vi "WKLXF25 Get Part Information 3.0.vi"(8 "error in":errorcluster, 11 "PLC Tags":T2={"Serial Number"={"Tag Name"="S060.PXI.Signals.PlltData.SN", "Network Path"="172.15.51.1,1,0", "use opc"=FALSE, "DataSocket Reference"={"CWDSLib._DCWDataSocket"=refnum, "CWDSLib._DCWData"=refnum, "OnDataUpdated"=0, "OnStatusUpdated"=0}}, "Pallet Number"={"Tag Name"="S060.PXI.Signals.PlltData.SN", "Network Path"="172.15.51.1,1,0", "use opc"=FALSE, "DataSocket Reference"={"CWDSLib._DCWDataSocket"=refnum, "CWDSLib._DCWData"=refnum, "OnDataUpdated"=0, "OnStatusUpdated"=0}}, "Inalfa Part Number"={"Tag Name"="S060.PXI.Signals.PlltData.SN", "Network Path"="172.15.51.1,1,0", "use opc"=FALSE, "DataSocket Reference"={"CWDSLib._DCWDataSocket"=refnum, "CWDSLib._DCWData"=refnum, "OnDataUpdated"=0, "OnStatusUpdated"=0}}, "Shade Color"={"Tag Name"="S060.PXI.Signals.PlltData.SN", "Network Path"="172.15.51.1,1,0", "use opc"=FALSE, "DataSocket Reference"={"CWDSLib._DCWDataSocket"=refnum, "CWDSLib._DCWData"=refnum, "OnDataUpdated"=0, "OnStatusUpdated"=0}}, "Model Type"={"Tag Name"="S060.PXI.Signals.PlltData.SN", "Network Path"="172.15.51.1,1,0", "use opc"=FALSE, "DataSocket Reference"={"CWDSLib._DCWDataSocket"=refnum, "CWDSLib._DCWData"=refnum, "OnDataUpdated"=0, "OnStatusUpdated"=0}}, "Customer Number"={"Tag Name"="S060.PXI.Signals.PlltData.SN", "Network Path"="172.15.51.1,1,0", "use opc"=FALSE, "DataSocket Reference"={"CWDSLib._DCWDataSocket"=refnum, "CWDSLib._DCWData"=refnum, "OnDataUpdated"=0, "OnStatusUpdated"=0}}, "Part History Number"={"Tag Name"="S060.PXI.Signals.PlltData.SN", "Network Path"="172.15.51.1,1,0", "use opc"=FALSE, "DataSocket Reference"={"CWDSLib._DCWDataSocket"=refnum, "CWDSLib._DCWData"=refnum, "OnDataUpdated"=0, "OnStatusUpdated"=0}}, "Shade 1 Barcode"={"Tag Name"="S060.PXI.Signals.PlltData.SN", "Network Path"="172.15.51.1,1,0", "use opc"=FALSE, "DataSocket Reference"={"CWDSLib._DCWDataSocket"=refnum, "CWDSLib._DCWData"=refnum, "OnDataUpdated"=0, "OnStatusUpdated"=0}}, "Shade 2 Barcode"={"Tag Name"="S060.PXI.Signals.PlltData.SN", "Network Path"="172.15.51.1,1,0", "use opc"=FALSE, "DataSocket Reference"={"CWDSLib._DCWDataSocket"=refnum, "CWDSLib._DCWData"=refnum, "OnDataUpdated"=0, "OnStatusUpdated"=0}}, "Manual Serial Number"={"Tag Name"="S060.PXI.Signals.PlltData.SN", "Network Path"="172.15.51.1,1,0", "use opc"=FALSE, "DataSocket Reference"={"CWDSLib._DCWDataSocket"=refnum, "CWDSLib._DCWData"=refnum, "OnDataUpdated"=0, "OnStatusUpdated"=0}}, "Manual Inalfa Part Number"={"Tag Name"="S060.PXI.Signals.PlltData.SN", "Network Path"="172.15.51.1,1,0", "use opc"=FALSE, "DataSocket Reference"={"CWDSLib._DCWDataSocket"=refnum, "CWDSLib._DCWData"=refnum, "OnDataUpdated"=0, "OnStatusUpdated"=0}}, "Manual Shade Color"={"Tag Name"="S060.PXI.Signals.PlltData.SN", "Network Path"="172.15.51.1,1,0", "use opc"=FALSE, "DataSocket Reference"={"CWDSLib._DCWDataSocket"=refnum, "CWDSLib._DCWData"=refnum, "OnDataUpdated"=0, "OnStatusUpdated"=0}}, "Manual Model Type"={"Tag Name"="S060.PXI.Signals.PlltData.SN", "Network Path"="172.15.51.1,1,0", "use opc"=FALSE, "DataSocket Reference"={"CWDSLib._DCWDataSocket"=refnum, "CWDSLib._DCWData"=refnum, "OnDataUpdated"=0, "OnStatusUpdated"=0}}, "Manual Customer Number"={"Tag Name"="S060.PXI.Signals.PlltData.SN", "Network Path"="172.15.51.1,1,0", "use opc"=FALSE, "DataSocket Reference"={"CWDSLib._DCWDataSocket"=refnum, "CWDSLib._DCWData"=refnum, "OnDataUpdated"=0, "OnStatusUpdated"=0}}, "Manual Part History Number"={"Tag Name"="S060.PXI.Signals.PlltData.SN", "Network Path"="172.15.51.1,1,0", "use opc"=FALSE, "DataSocket Reference"={"CWDSLib._DCWDataSocket"=refnum, "CWDSLib._DCWData"=refnum, "OnDataUpdated"=0, "OnStatusUpdated"=0}}} {"Manual Part History Number"."DataSocket Reference"."OnStatusUpdated" format="%.0x"; "Manual Part History Number"."DataSocket Reference"."OnDataUpdated" format="%.0x"; "Manual Customer Number"."DataSocket Reference"."OnStatusUpdated" format="%.0x"; "Manual Customer Number"."DataSocket Reference"."OnDataUpdated" format="%.0x"; "Manual Model Type"."DataSocket Reference"."OnStatusUpdated" format="%.0x"; "Manual Model Type"."DataSocket Reference"."OnDataUpdated" format="%.0x"; "Manual Shade Color"."DataSocket Reference"."OnStatusUpdated" format="%.0x"; "Manual Shade Color"."DataSocket Reference"."OnDataUpdated" format="%.0x"; "Manual Inalfa Part Number"."DataSocket Reference"."OnStatusUpdated" format="%.0x"; "Manual Inalfa Part Number"."DataSocket Reference"."OnDataUpdated" format="%.0x"; "Manual Serial Number"."DataSocket Reference"."OnStatusUpdated" format="%.0x"; "Manual Serial Number"."DataSocket Reference"."OnDataUpdated" format="%.0x"; "Shade 2 Barcode"."DataSocket Reference"."OnStatusUpdated" format="%.0x"; "Shade 2 Barcode"."DataSocket Reference"."OnDataUpdated" format="%.0x"; "Shade 1 Barcode"."DataSocket Reference"."OnStatusUpdated" format="%.0x"; "Shade 1 Barcode"."DataSocket Reference"."OnDataUpdated" format="%.0x"; "Part History Number"."DataSocket Reference"."OnStatusUpdated" format="%.0x"; "Part History Number"."DataSocket Reference"."OnDataUpdated" format="%.0x"; "Customer Number"."DataSocket Reference"."OnStatusUpdated" format="%.0x"; "Customer Number"."DataSocket Reference"."OnDataUpdated" format="%.0x"; "Model Type"."DataSocket Reference"."OnStatusUpdated" format="%.0x"; "Model Type"."DataSocket Reference"."OnDataUpdated" format="%.0x"; "Shade Color"."DataSocket Reference"."OnStatusUpdated" format="%.0x"; "Shade Color"."DataSocket Reference"."OnDataUpdated" format="%.0x"; "Inalfa Part Number"."DataSocket Reference"."OnStatusUpdated" format="%.0x"; "Inalfa Part Number"."DataSocket Reference"."OnDataUpdated" format="%.0x"; "Pallet Number"."DataSocket Reference"."OnStatusUpdated" format="%.0x"; "Pallet Number"."DataSocket Reference"."OnDataUpdated" format="%.0x"; "Serial Number"."DataSocket Reference"."OnStatusUpdated" format="%.0x"; "Serial Number"."DataSocket Reference"."OnDataUpdated" format="%.0x"}) -> (0 "error out":errorcluster, 2 "Good Data?":bool, 3 "part info":T1)   [LabVIEW 2018]
uses:
  02.Type Def's/station plc read string tags.ctl
  05.UserVI's/type defs/plc path and tag.ctl
  <vilib>/Platform/dataskt.llb/DataSocket Reference Type.ctl
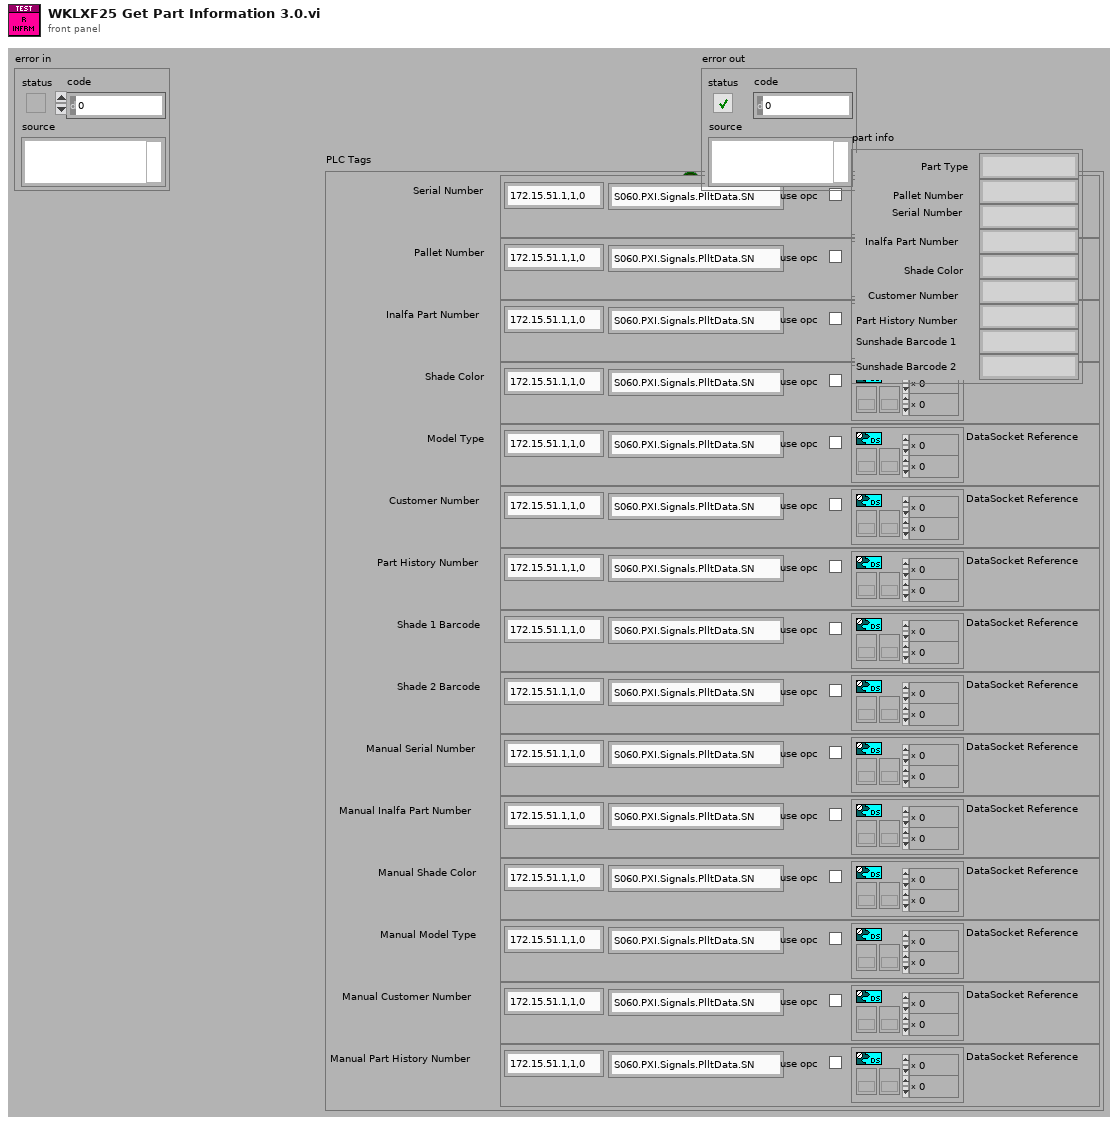
[diagram p1: front panel]
types:
  T1 = cluster{"Serial Number":string, "Pallet Number":string, "Inalfa Part Number":string, "Part Type":string, "Shade Color":string, "Customer Number":string, "Part History Number":string, "Sunshade Barcode 2":string, "Sunshade Barcode 1":string}
  T2 = typedef "station plc read string tags.ctl" = cluster{"Serial Number":T3, "Pallet Number":T3, "Inalfa Part Number":T3, "Shade Color":T3, "Model Type":T3, "Customer Number":T3, "Part History Number":T3, "Shade 1 Barcode":T3, "Shade 2 Barcode":T3, "Manual Serial Number":T3, "Manual Inalfa Part Number":T3, "Manual Shade Color":T3, "Manual Model Type":T3, "Manual Customer Number":T3, "Manual Part History Number":T3}
  T3 = typedef "plc path and tag.ctl" = cluster{"Tag Name":string, "Network Path":string, "use opc":bool, "DataSocket Reference":T4}
  T4 = typedef "DataSocket Reference Type.ctl" = cluster{"CWDSLib._DCWDataSocket":refnum<k7>, "CWDSLib._DCWData":refnum<k7>, "OnDataUpdated":u32, "OnStatusUpdated":u32}
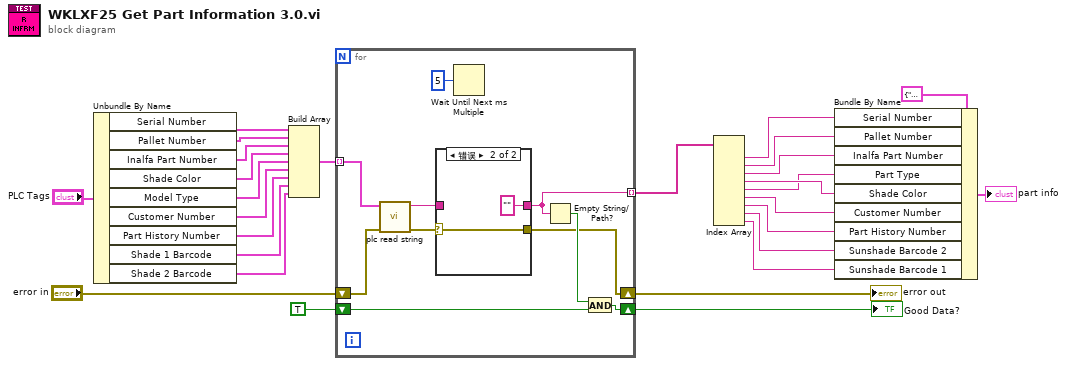
[diagram p0: block diagram]
diagram:
  n1 = Unbundle By Name("PLC Tags") -> ("Serial Number"=w23:T3, "Pallet Number"=w22:T3, "Inalfa Part Number"=w21:T3, "Shade Color"=w20:T3, "Model Type"=w19:T3, "Customer Number"=w18:T3, "Part History Number"=w17:T3, "Shade 1 Barcode"=w16:T3, "Shade 2 Barcode"=w15:T3)
  n2 = Build Array(w23, w22, w21, w20, w19, w18, w17, w16, w15) -> (w14:T3[])
  n3 = for {
    tunnel: [w37] -> w25 mode=indexing
    shift-right: [w35] -> w26
    shift-left: TRUE -> [w34]
    tunnel: w14 -> [w32] mode=indexing
    shift-right: [w33] -> w12
    shift-left: "error in" -> [w31]
    n4 = call "plc read string.vi"("error in"=w31, "addr,tag"=w32) -> ("error out"=w29:errorcluster, "Data"=w30:string)  [unwired: 8 in]
    n5 = case shown="错误" w29 {
      selector: w29 -> [w38 w40]
      tunnel: w30 -> [w39 _]
      tunnel: [w39 ""] -> w37
      tunnel: [w38 w40] -> w33
      frame No Error {
      }
      frame Error {
      }
    }
    n6 = Wait Until Next ms Multiple(millisecond multiple=u32 5) -> ()  [unwired: 1 out]
    n7 = Empty String/Path?(string/path=w37) -> (empty?=w36:bool)
    n8 = And(x=w36, y=w34) -> (x .and. y?=w35:bool)
  }
  "Good Data?" <- w26
  "error out" <- w12
  n9 = Index Array(array=w25) -> (element #1=w9:string, element #2=w8:string, element #3=w7:string, element #4=w6:string, element #5=w5:string, element #6=w4:string, element #7=w3:string, element #8=w2:string, element #9=w1:string)  [unwired: 9 in]
  n10 = Bundle By Name(cluster=T1 {"Serial Number"="", "Pallet Number"="", "Inalfa Part Number"="", "Part Type"="", "Shade Color"="", "Customer Number"="", "Part History Number"="", "Sunshade Barcode 2"="", "Sunshade Barcode 1"=""} ("part info"), "Serial Number"=w9, "Pallet Number"=w8, "Inalfa Part Number"=w7, "Part Type"=w5, "Shade Color"=w6, "Customer Number"=w4, "Part History Number"=w3, "Sunshade Barcode 2"=w2, "Sunshade Barcode 1"=w1) -> (→"part info":T1)
